vi "Write Tick.vi"(10 "Tick":u32, 11 "PID Timing Estimation in":refnum<class "PID Timing Estimation.lvclass">) -> (3 "PID Timing Estimation out":refnum<class "PID Timing Estimation.lvclass">)   [LabVIEW 2019, in "control.lvlib" / "PID Timing Estimation.lvclass"]
uses:
  PID Timing Estimation.lvclass
  PID Timing Estimation.lvclass/PID Timing Estimation.ctl
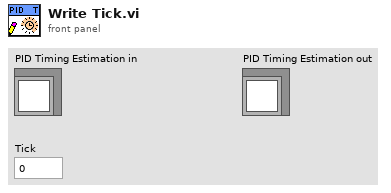
[diagram p1: front panel]
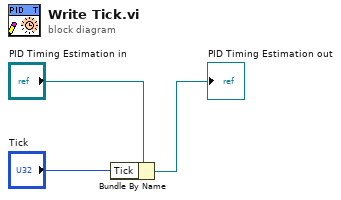
[diagram p0: block diagram]
diagram:
  n1 = Bundle By Name(cluster="PID Timing Estimation in", "Tick"="Tick") -> (→"PID Timing Estimation out":refnum<class "PID Timing Estimation.lvclass">)
